vi "publishTelemetry.vi"(8 "error in (no error)":errorcluster, 11 "Model in":refnum<class "Model.lvclass">) -> (0 "error out":errorcluster, 3 "Model out":refnum<class "Model.lvclass">)   [LabVIEW 2016, in "Model.lvclass"]
uses:
  Model.lvclass
  Model.lvclass/Model.ctl
  Telemetry/Telemetry.lvclass
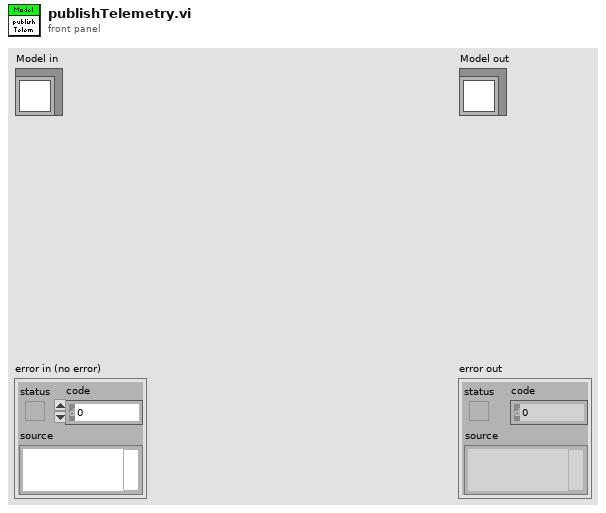
[diagram p1: front panel]
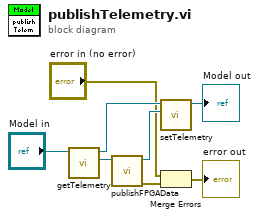
[diagram p0: block diagram]
diagram:
  n1 = call "getTelemetry.vi"("Model in"="Model in") -> ("Telemetry"=w7:refnum<class "Telemetry.lvclass">, "Model out"=w6:refnum<class "Model.lvclass">)  [unwired: 9 in]
  n2 = call "publishFPGAData.vi"("Telemetry in"=w7) -> ("error out"=w3:errorcluster, "Telemetry out"=w5:refnum<class "Telemetry.lvclass">)  [unwired: 9 in]
  n3 = call "setTelemetry.vi"("Telemetry"=w5, "Model in"=w6) -> ("Model out"=→"Model out":refnum<class "Model.lvclass">)  [unwired: 9 in]
  n4 = Merge Errors("error in (no error)", w3) -> (→"error out":errorcluster)
